vi "Create DI Scope Page.vi"(8 "error in (no error)":errorcluster, 11 "Section Ptr":T3 format="%.0x") -> (0 "error out":errorcluster, 3 "Parent Ref out":T3 format="%.0x")   [LabVIEW 2016, in "DCM System Explorer.lvlib"]
uses:
  DCM System Explorer.lvlib
  <vilib>/NI Veristand/Custom Device API/Custom Device Item Ref.ctl
  <vilib>/Powertrain Controls/Device Drivers/DCM/Rev0/FPGA/DI - ADC Signals.ctl
  <vilib>/Powertrain Controls/Device Drivers/DCM/DI/FPGA/Capture Event.ctl
  <vilib>/NI Veristand/Custom Device API/Custom Device Channel Type.ctl
  <vilib>/NI Veristand/Custom Device API/Custom Device Waveform.ctl
  <vilib>/NI Veristand/Custom Device API/Custom Device Waveform DataType.ctl
  Shared/DCM Constants and GUIDs.vi
  DCM Shared.lvlib
  <vilib>/NI VeriStand/Custom Device API/Custom Device API.lvlib
  <vilib>/Powertrain Controls/Device Drivers/DCM/Rev0/FPGA/DCM - FPGA.lvlib
  <vilib>/Powertrain Controls/Device Drivers/DCM/DI/FPGA/DCM - FPGA - DI.lvlib
panel:
  in  "Capture Event":T1
  in  "DI ADC 1":T2
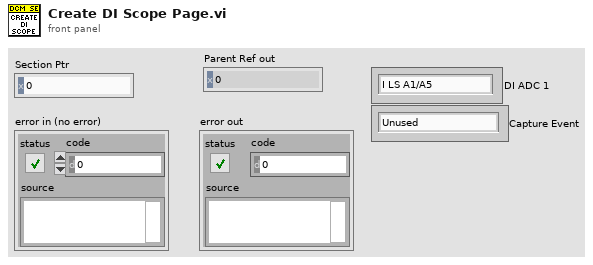
[diagram p1: front panel]
types:
  T1 = typedef "DCM - FPGA - DI.lvlib/Capture Event.ctl" = enum8{"Unused", "Injector A1", "Injector A2", "Injector A3", "Injector A4", "Injector A5", "Injector A6", "Injector A7", "Injector A8/PumpA", "Injector B1", "Injector B2", "Injector B3", "Injector B4", "Injector B5", "Injector B6", "Injector B7", "Injector B8/PumpB", "User OS", "Diff IO 1", "Diff IO 2", "Diff IO 3", "Diff IO 4", "Diff IO 5", "Diff IO 6", "Diff IO 7", "Diff IO 8", "Aux 1", "Aux 2", "Aux 3", "Aux 4", "Aux 5", "Aux 6", "Aux 7", "Aux 8", "Aux 9", "Aux 10", "Aux 11", "Aux 12", "Aux 13", "Aux 14", "Aux 15", "Aux 16"}
  T2 = typedef "DCM - FPGA.lvlib/DI - ADC Signals.ctl" = enum8{"I LS A1/A5", "I LS A2/A6", "I LS A3/A7", "I LS A4", "I LS A8/PumpA", "V PZ A1", "V PZ A2", "V PZ A3", "V PZ A4", "V S A1", "V S A2", "V S A3", "V S A4", "V S A5", "V S A6", "V S A7", "V S A8", "V Pump A", "V Secondary A1A2", "V Secondary A3A4", "V Ext HV A", "------------------------ ", "I LS B1/B5", "I LS B2/B6", "I LS B3/B7", "I LS B4", "I LS B8/PumpB", "V PZ B1", "V PZ B2", "V PZ B3", "V PZ B4", "V S B1", "V S B2", "V S B3", "V S B4", "V S B5", "V S B6", "V S B7", "V S B8", "V Pump B", "V Secondary B1B2", "V Secondary B3B4", "V Ext HV B", "-------------------------  ", "AI 1", "AI 2", "AI 3", "AI 4", "AI 5", "AI 6", "AI 7", "AI 8", "AI 9", "AI 10", "AI 11", "AI 12", "-------------------------   ", "V DRVP"}
  T3 = typedef "Custom Device API.lvlib/Custom Device Item Ref.ctl" = u64
  T4 = typedef "Custom Device API.lvlib/Custom Device Channel Type.ctl" = enum16{"Input", "Output"}
  T5 = typedef "DCM Shared.lvlib/Channel.ctl" = cluster{"Name":string, "Units":string, "Default":dbl, "Description":string}
  T6 = typedef "Custom Device API.lvlib/Custom Device Waveform DataType.ctl" = enum16{"Double", "Complex Double"}
  T7 = typedef "Custom Device API.lvlib/Custom Device Waveform.ctl" = cluster{"Data Type":T6, "Units":string}
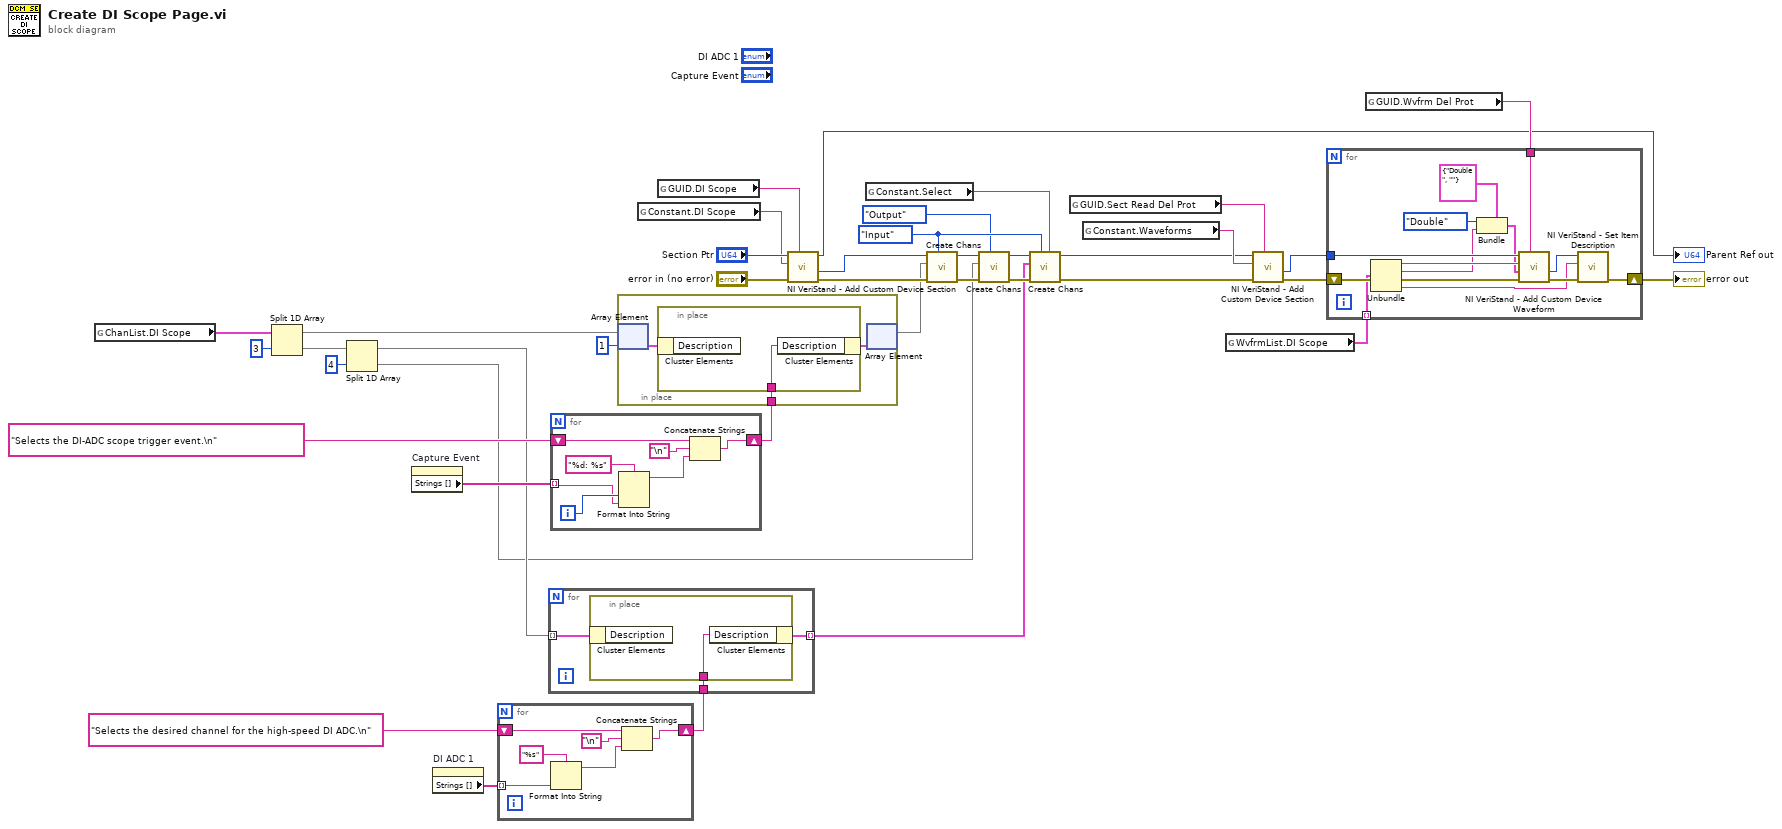
[diagram p0: block diagram]
diagram:
  w8 = Custom_Device_Channel_Type."Input" ("Type")
  n1 = global read "DCM Constants and GUIDs.vi" "ChanList.DI Scope"() -> (w21:T5[])
  n2 = Split 1D Array(array=w21, index=3) -> (first subarray=w15:T5[], second subarray=w4:T5[])
  n3 = Split 1D Array(array=w4, index=4) -> (first subarray=w2:T5[], second subarray=w1:T5[])
  n4 = property on="Capture Event" class="Enum (strict)"() -> ("Strings []"=w22:string[])  [unwired: 2 in, 2 out]
  n5 = property on="DI ADC 1" class="Enum (strict)"() -> ("Strings []"=w27:string[])  [unwired: 2 in, 2 out]
  n6 = for {
    tunnel: w27 -> [w40] mode=indexing
    shift-right: [w41] -> w25
    shift-left: "Selects the desired channel for the high-speed DI ADC.\n" ("format string") -> [w44]
    n7 = Format Into String(format string="%s", w40) -> (resulting string=w43:string)  [unwired: 2 in, 1 out]
    n8 = Concatenate Strings(w44, "\n", w43) -> (w41:string)
  }
  n9 = for {
    tunnel: w2 -> [w48] mode=indexing
    tunnel: w25 -> [w47]
    tunnel: [w46] -> w6 mode=indexing
    n10 = in-place {
      in-place-border: w47 -> [w49]
      n11 = in-place-cluster #1(w48) -> ()  [unwired: 1 out]
      n12 = in-place-cluster #1("Description"=w49) -> (w46:T5)
    }
  }
  n13 = for {
    tunnel: w22 -> [w50] mode=indexing
    shift-right: [w52] -> w24
    shift-left: "Selects the DI-ADC scope trigger event.\n" ("format string") -> [w55]
    i -> [w51]
    n14 = Format Into String(format string="%d: %s", w51, w50) -> (resulting string=w54:string)  [unwired: 2 in, 1 out]
    n15 = Concatenate Strings(w55, "\n", w54) -> (w52:string)
  }
  n16 = in-place {
    in-place-border: w24 -> [w59]
    n17 = in-place-array #2(w15, 1) -> (w58:T5)
    n18 = in-place {
      in-place-border: w59 -> [w60]
      n19 = in-place-cluster #3(w58) -> ()  [unwired: 1 out]
      n20 = in-place-cluster #3("Description"=w60) -> (w57:T5)
    }
    n21 = in-place-array #2(w57) -> (w14:T5[])  [unwired: 1 out]
  }
  n22 = global read "DCM Constants and GUIDs.vi" "Constant.DI Scope"() -> (w30:string)
  n23 = global read "DCM Constants and GUIDs.vi" "GUID.DI Scope"() -> (w29:string)
  n24 = call <vilib>:"NI VeriStand - Add Custom Device Section.vi"("GUID (Default Section)"=w29, "error in (no error)"="error in (no error)", "Section Name"=w30, "Parent Ref in"="Section Ptr") -> ("error out"=w19:errorcluster, "Section Ptr"=w18:T3, "Parent Ref out"=→"Parent Ref out":T3)  [unwired: 4 in, 1 out]
  n25 = global read "DCM Constants and GUIDs.vi" "Constant.Select"() -> (w7:string)
  n26 = call "Create Chans.vi"("Type"=w8, "error in (no error)"=w19, "Channels"=w14, "Section Ptr"=w18) -> ("error out"=w16:errorcluster, "Section Ptr dup"=w17:T3)  [unwired: 4 in, 2 out]
  n27 = call "Create Chans.vi"("Type"=Custom_Device_Channel_Type."Output", "error in (no error)"=w16, "Channels"=w1, "Section Ptr"=w17) -> ("error out"=w10:errorcluster, "Section Ptr dup"=w12:T3)  [unwired: 4 in, 2 out]
  n28 = call "Create Chans.vi"("New Section Name (none)"=w7, "Type"=w8, "error in (no error)"=w10, "Channels"=w6, "Section Ptr"=w12) -> ("error out"=w9:errorcluster, "Section Ptr dup"=w11:T3)  [unwired: 3 in, 2 out]
  n29 = global read "DCM Constants and GUIDs.vi" "GUID.Sect Read Del Prot"() -> (w34:string)
  n30 = global read "DCM Constants and GUIDs.vi" "Constant.Waveforms"() -> (w35:string)
  n31 = global read "DCM Constants and GUIDs.vi" "WvfrmList.DI Scope"() -> (w37:T5[])
  n32 = call <vilib>:"NI VeriStand - Add Custom Device Section.vi"("GUID (Default Section)"=w34, "error in (no error)"=w9, "Section Name"=w35, "Parent Ref in"=w11) -> ("error out"=w36:errorcluster, "Section Ptr"=w33:T3)  [unwired: 4 in, 2 out]
  n33 = global read "DCM Constants and GUIDs.vi" "GUID.Wvfrm Del Prot"() -> (w38:string)
  n34 = for {
    tunnel: w33 -> [w73]
    tunnel: w38 -> [w71]
    shift-right: [w68] -> w39
    shift-left: w36 -> [w72]
    tunnel: w37 -> [w65] mode=indexing
    n35 = Unbundle(w65) -> ("Name"=w64:string, "Units"=w62:string, "Description"=w61:string)  [unwired: 1 out]
    n36 = Bundle(cluster=T7 {"Data Type"=enum."Double", "Units"=""} ("Waveform"), "Data Type"=Custom_Device_Waveform_DataType."Double", "Units"=w62) -> (w63:T7)
    n37 = call <vilib>:"NI VeriStand - Add Custom Device Waveform.vi"("GUID (Default Waveform)"=w71, "error in (no error)"=w72, "Waveform"=w63, "Waveform Name"=w64, "Parent Ref in"=w73) -> ("error out"=w70:errorcluster, "Waveform Ref"=w69:T3)  [unwired: 3 in, 2 out]
    n38 = call <vilib>:"NI VeriStand - Set Item Description.vi"("error in (no error)"=w70, "Description"=w61, "Item Ref in"=w69) -> ("error out"=w68:errorcluster)  [unwired: 6 in, 2 out]
  }
  "error out" <- w39
